vi "Undo.vi"(8 "error in (no error)":errorcluster, 11 "Picture.lvclass in":refnum<class "Picture.lvclass">) -> (0 "error out":errorcluster, 2 "Removed Object":refnum<class "Graphics Object.lvclass">, 3 "Picture.lvclass out":refnum<class "Picture.lvclass">)   [LabVIEW 2020, in "Picture.lvclass"]
doc: "Removes the last added object from a picture"
uses:
  Picture.lvclass
  Graphics Object/Graphics Object.lvclass
  Picture.lvclass/Picture.ctl
  Empty/Empty.lvclass
  D:/Git/Labview-Libraries/Tools/Drawing Tool Folder/Graphics Object/Graphics Object.lvclass
panel:
  # "expressionflow.com"
  # "Copyright (c) 2008 Tomi Maila. All rights reserved."
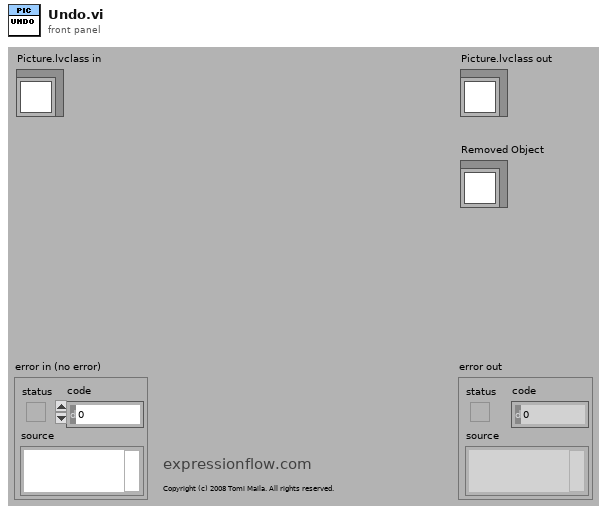
[diagram p1: front panel]
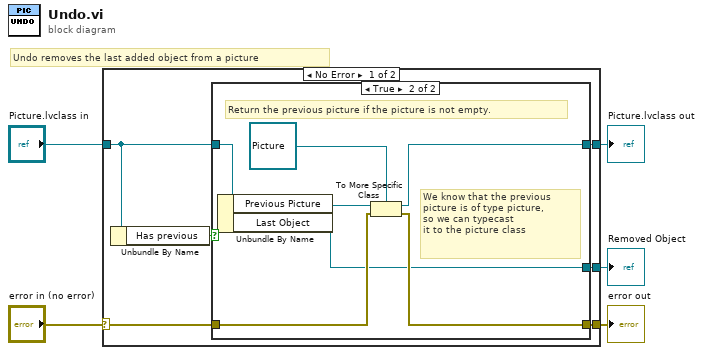
[diagram p0: block diagram]
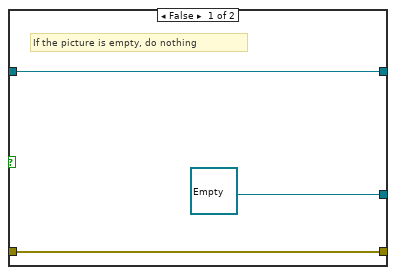
[diagram p2: hidden frame]
diagram:
  # "Undo removes the last added object from a picture"
  n1 = case shown="No Error" "error in (no error)" {
    selector: "error in (no error)" -> [w10 w22]
    tunnel: [w9 w22] -> w4
    tunnel: [w11 w23] -> w1
    tunnel: "Picture.lvclass in" -> [w7 w23]
    tunnel: [w6 _] -> w2
    frame No Error {
      n2 = Unbundle By Name(w7) -> ("Has previous"=w8:bool)
      n3 = case shown="True" w8 {
        tunnel: [w14 w21] -> w11
        tunnel: w10 -> [w12 w20]
        tunnel: [w12 w19] -> w9
        tunnel: w7 -> [w14 w18]
        tunnel: [refnum<class "Empty.lvclass"> refnum ("Empty.lvclass") w16] -> w6
        frame False {
          # "If the picture is empty, do nothing"
        }
        frame True {
          # "We know that the previous\npicture is of type picture,\nso we can typecast\nit to the picture class"
          # "Return the previous picture if the picture is not empty."
          n4 = Unbundle By Name(w18) -> ("Previous Picture"=w17:refnum<class "Graphics Object.lvclass">, "Last Object"=w16:refnum<class "Graphics Object.lvclass">)
          n5 = To More Specific Class(target class=refnum<class "Picture.lvclass"> refnum ("Picture.lvclass out"), reference=w17, error in=w20) -> (specific class reference=w21:refnum<class "Picture.lvclass">, error out=w19:errorcluster)
        }
      }
    }
    frame Error {
    }
  }
  "error out" <- w4
  "Picture.lvclass out" <- w1
  "Removed Object" <- w2
